vi "Digital Y.vi"(11 "Input Y":u16) -> ()   [LabVIEW 2015]
uses:
  <vilib>/rvi/eio/common/nirviEmuTemplateMethod_errors.vi
  <vilib>/eio/EIONode/EIONode.xnode
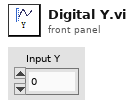
[diagram p1: front panel]
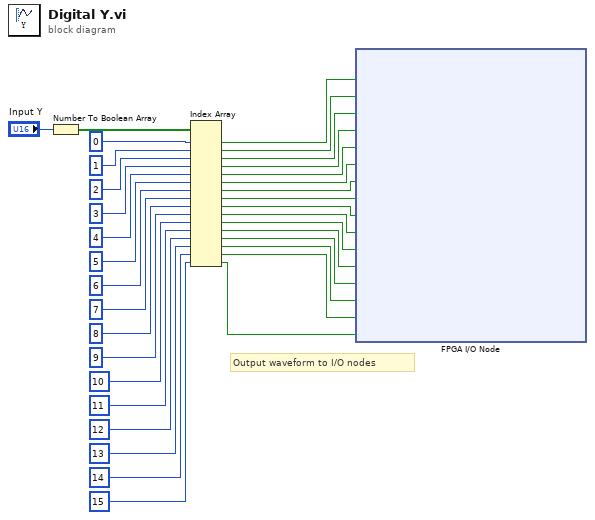
[diagram p0: block diagram]
diagram:
  # "Output waveform to I/O nodes"
  n1 = Number To Boolean Array(number="Input Y") -> (Boolean array=w33:bool[])
  n2 = Index Array(array=w33, index #1=0 ("index"), index #2=1 ("index"), index #3=2 ("index"), index #4=3 ("index"), index #5=4 ("index"), index #6=5 ("index"), index #7=6 ("index"), index #8=7 ("index"), index #9=8 ("index"), index #10=9 ("index"), index #11=10 ("index"), index #12=11 ("index"), index #13=12 ("index"), index #14=13 ("index"), index #15=14 ("index"), index #16=15 ("index")) -> (element #1=w17:bool, element #2=w18:bool, element #3=w19:bool, element #4=w20:bool, element #5=w21:bool, element #6=w22:bool, element #7=w23:bool, element #8=w24:bool, element #9=w25:bool, element #10=w26:bool, element #11=w27:bool, element #12=w28:bool, element #13=w29:bool, element #14=w30:bool, element #15=w31:bool, element #16=w32:bool)
  n3 = xnode "FPGA I/O Node"("IO Module\\DDCB_DIO8_WRITE"=w17, "IO Module\\DDCB_DIO9_WRITE"=w18, "IO Module\\DDCB_DIO10_WRITE"=w19, "IO Module\\DDCB_DIO11_WRITE"=w20, "IO Module\\DDCB_DIO12_WRITE"=w21, "IO Module\\DDCB_DIO13_WRITE"=w22, "IO Module\\DDCB_DIO14_WRITE"=w23, "IO Module\\DDCB_DIO15_WRITE"=w24, "IO Module\\DDCB_DIO16_WRITE"=w25, "IO Module\\DDCB_DIO17_WRITE"=w26, "IO Module\\DDCB_DIO18_WRITE"=w27, "IO Module\\DDCB_DIO19_WRITE"=w28, "IO Module\\DDCB_DIO20_WRITE"=w29, "IO Module\\DDCB_DIO21_WRITE"=w30, "IO Module\\DDCB_DIO22_WRITE"=w31, "IO Module\\DDCB_DIO23_WRITE"=w32) -> ()  [unwired: 16 in, 16 out]
